vi "copy.vi"(8 "error in (no error)":errorcluster, 10 "ScriptEventForCopy":refnum<class "ScriptEvent.lvclass">, 11 "RampUp in":refnum<class "RampUp.lvclass">) -> (0 "error out":errorcluster, 3 "RampUp Copy":refnum<class "RampUp.lvclass">)   [LabVIEW 2009, in "Tools.lvlib" / "Scripting.lvlib" / "RampUp.lvclass"]
uses:
  RampUp.lvclass
  ScriptEvent.lvclass
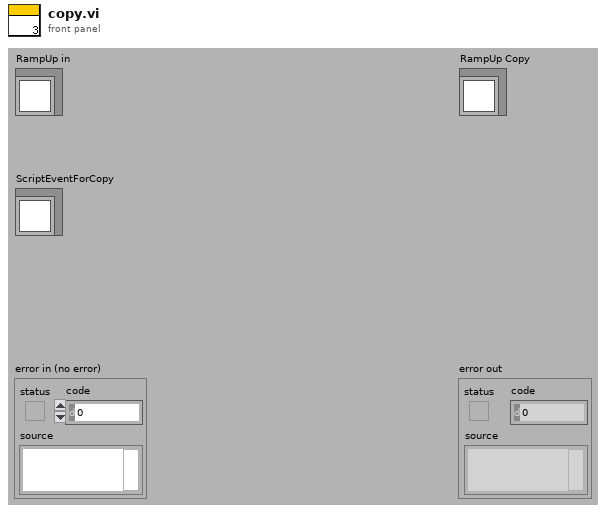
[diagram p1: front panel]
types:
  T1 = enum16{"changeValue", "pulse", "clock", "rampUp", "rampDown", "singleTone", "singleToneRamp", "playFile", "rf", "rfRamp"}
  T2 = enum16{"Initialise", "MOT", "Molasses", "Optical Pumping", "Magnetic Trap", "RF Cooling", "Manipulation", "Switch Off", "Absorption Imaging", "Fluorscence Imaging", "Shut Down"}
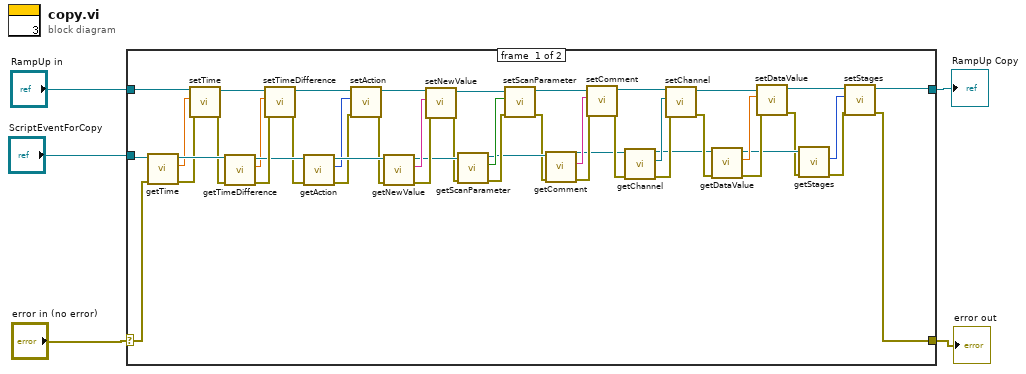
[diagram p0: block diagram]
diagram:
  n1 = case shown="No Error" "error in (no error)" {
    selector: "error in (no error)" -> [w6 w53]
    tunnel: "RampUp in" -> [w17 w54]
    tunnel: [w7 w54] -> w3
    tunnel: [w18 w53] -> w2
    tunnel: "ScriptEventForCopy" -> [w52 _]
    frame #0 {
      n2 = call "getTime.vi"("error in (no error)"=w6, "ScriptEvent.lvclass in"=w52) -> ("error out"=w50:errorcluster, "time"=w49:dbl, "ScriptEvent.lvclass out"=w51:refnum<class "ScriptEvent.lvclass">)  [unwired: 7 in]
      n3 = call "setTime.vi"("error in (no error)"=w50, "time"=w49, "ScriptEvent.lvclass in"=w17) -> ("error out"=w48:errorcluster, "ScriptEvent.lvclass out"=w15:refnum<class "RampUp.lvclass">)  [unwired: 7 in]
      n4 = call "getTimeDifference.vi"("error in (no error)"=w48, "ScriptEvent.lvclass in"=w51) -> ("error out"=w47:errorcluster, "time difference"=w16:dbl, "ScriptEvent.lvclass out"=w46:refnum<class "ScriptEvent.lvclass">)  [unwired: 7 in]
      n5 = call "setTimeDifference.vi"("error in (no error)"=w47, "time difference"=w16, "ScriptEvent.lvclass in"=w15) -> ("error out"=w45:errorcluster, "ScriptEvent.lvclass out"=w14:refnum<class "RampUp.lvclass">)  [unwired: 7 in]
      n6 = call "getAction.vi"("error in (no error)"=w45, "ScriptEvent.lvclass in"=w46) -> ("error out"=w43:errorcluster, "action"=w42:T1, "ScriptEvent.lvclass out"=w44:refnum<class "ScriptEvent.lvclass">)  [unwired: 7 in]
      n7 = call "setAction.vi"("error in (no error)"=w43, "action"=w42, "ScriptEvent.lvclass in"=w14) -> ("error out"=w41:errorcluster, "ScriptEvent.lvclass out"=w13:refnum<class "RampUp.lvclass">)  [unwired: 7 in]
      n8 = call "getNewValue.vi"("error in (no error)"=w41, "ScriptEvent.lvclass in"=w44) -> ("error out"=w40:errorcluster, "newValue"=w39:string, "ScriptEvent.lvclass out"=w38:refnum<class "ScriptEvent.lvclass">)  [unwired: 7 in]
      n9 = call "setNewValue.vi"("error in (no error)"=w40, "newValue"=w39, "ScriptEvent.lvclass in"=w13) -> ("error out"=w37:errorcluster, "ScriptEvent.lvclass out"=w12:refnum<class "RampUp.lvclass">)  [unwired: 7 in]
      n10 = call "getScanParameter.vi"("error in (no error)"=w37, "ScriptEvent.lvclass in"=w38) -> ("error out"=w35:errorcluster, "scanParameter"=w36:bool, "ScriptEvent.lvclass out"=w34:refnum<class "ScriptEvent.lvclass">)  [unwired: 7 in]
      n11 = call "setScanParameter.vi"("error in (no error)"=w35, "scanParameter"=w36, "ScriptEvent.lvclass in"=w12) -> ("error out"=w33:errorcluster, "ScriptEvent.lvclass out"=w11:refnum<class "RampUp.lvclass">)  [unwired: 7 in]
      n12 = call "getComment.vi"("error in (no error)"=w33, "ScriptEvent.lvclass in"=w34) -> ("error out"=w32:errorcluster, "comment"=w31:string, "ScriptEvent.lvclass out"=w29:refnum<class "ScriptEvent.lvclass">)  [unwired: 7 in]
      n13 = call-dynamic "setComment.vi"("error in (no error)"=w32, "comment"=w31, "RampEvent.lvclass in"=w11) -> ("error out"=w30:errorcluster, "RampEvent.lvclass out"=w10:refnum<class "RampUp.lvclass">)  [unwired: 7 in]
      n14 = call-dynamic "getChannel.vi"("error in (no error)"=w30, "ScriptEvent.lvclass in"=w29) -> ("error out"=w28:errorcluster, "Channel.lvclass"=w27:refnum<class "Channel.lvclass">, "ScriptEvent.lvclass out"=w25:refnum<class "ScriptEvent.lvclass">)  [unwired: 7 in]
      n15 = call-dynamic "setChannel.vi"("error in (no error)"=w28, "Channel.lvclass"=w27, "RampEvent.lvclass in"=w10) -> ("error out"=w26:errorcluster, "RampEvent.lvclass out"=w9:refnum<class "RampUp.lvclass">)  [unwired: 7 in]
      n16 = call "getDataValue.vi"("error in (no error)"=w26, "ScriptEvent.lvclass in"=w25) -> ("error out"=w24:errorcluster, "dataValue"=w23:dbl, "ScriptEvent.lvclass out"=w22:refnum<class "ScriptEvent.lvclass">)  [unwired: 7 in]
      n17 = call "setDataValue.vi"("error in (no error)"=w24, "dataValue"=w23, "ScriptEvent.lvclass in"=w9) -> ("error out"=w21:errorcluster, "ScriptEvent.lvclass out"=w8:refnum<class "RampUp.lvclass">)  [unwired: 7 in]
      n18 = call "getStages.vi"("error in (no error)"=w21, "ScriptEvent.lvclass in"=w22) -> ("error out"=w20:errorcluster, "Stage"=w19:T2)  [unwired: 7 in, 1 out]
      n19 = call-dynamic "setStages.vi"("error in (no error)"=w20, "Stage"=w19, "RampEvent.lvclass in"=w8) -> ("error out"=w18:errorcluster, "RampEvent.lvclass out"=w7:refnum<class "RampUp.lvclass">)  [unwired: 7 in]
    }
    frame #1 {
    }
  }
  "error out" <- w2
  "RampUp Copy" <- w3
